vi "Close.vi"(8 "error in (no error)":errorcluster, 11 "Base CFG in":refnum<class "Scope PXI Base CFG.lvclass">) -> (0 "error out":errorcluster, 3 "Base CFG out":refnum<class "Scope PXI Base CFG.lvclass">)   [LabVIEW 2023, in "Scope PXI Base CFG.lvclass"]
uses:
  Scope PXI Base CFG.lvclass
  Scope PXI Base CFG.lvclass/Scope PXI Base CFG.ctl
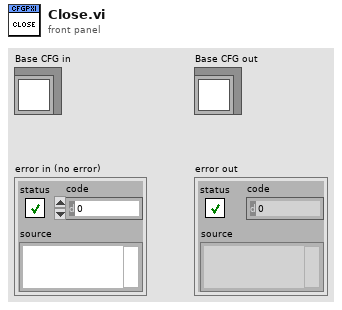
[diagram p1: front panel]
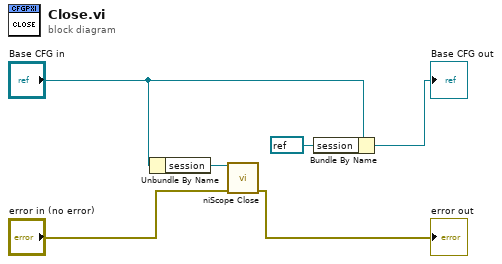
[diagram p0: block diagram]
diagram:
  n1 = Unbundle By Name("Base CFG in") -> ("session"=w6:refnum<k15>)
  n2 = call <instrlib>:"niScope Close.vi"("instrument handle"=w6, "error in"="error in (no error)") -> ("error out"=→"error out":errorcluster)  [unwired: 13 in]
  n3 = Bundle By Name(cluster="Base CFG in", "session"=refnum<k15> refnum) -> (→"Base CFG out":refnum<class "Scope PXI Base CFG.lvclass">)
